vi "Laser Fine Cutting.vi"(0 "configuration file path":path=path "C:/Users/admin/OneDrive/文档/Inlafa.CCV254.MES/System/All Config.ini" caption="配置文件的路径", 1 "fine cutting msic":T1) -> ()   [LabVIEW 2014]
uses:
  Ctl.xio/fine cutting msic ctl.ctl
  SubVIS.xio/DataSocket/DataSocket_Tags.ctl
  Ctl.xio/part type.ctl
  SubVIS.xio/Creat Write List VI's/DefCtrl/Station.ctl
  SubVIS.xio/DataSocket/Write PLC Vars/Write String Var in.vi
  <vilib>/Utility/file.llb/Read From Spreadsheet File (string).vi
  SubVIS.xio/DataSocket/Write PLC Vars/Write Bool Var in.vi
  SubVIS.xio/DataSocket/Read PLC Vars/Read String Var.vi
  SubVIS.xio/DataSocket/Write PLC Vars/Write Dbl Var in.vi
  SubVIS.xio/DataSocket/Read PLC Vars/Read Bool Var.vi
  SubVIS.xio/DataSocket/Read PLC Vars/Read U32 Var.vi
panel:
  in  "SQL information":string
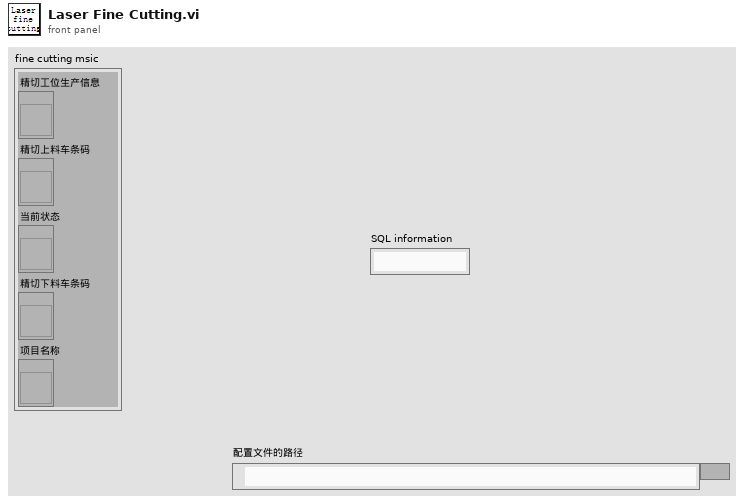
[diagram p1: front panel]
types:
  T1 = cluster{"精切工位生产信息":refnum<vi>, "精切上料车条码":refnum<vi>, "当前状态":refnum<vi>, "精切下料车条码":refnum<vi>, "项目名称":refnum<vi>}
  T2 = typedef "Station.ctl" = enum16{"粗切工位", "热处理工位", "精切工位", "PDF焊接工位", "打凹点预载力工位", "收卷工位", "EOL工位"}
  T3 = typedef "fine cutting msic ctl.ctl" = cluster{"configuration file path":path, "DsOut":T4[], "Hopper in car information":cluster{"Hopper car code":string, "Hopper car No":string, "plate No":string}, "pallet.produced number":i32, "SQL information":string, "Database":string[], "Serial number":i32, "database path":path, "fine cutting msic":cluster{"精切工位生产信息":refnum<vi>, "精切上料车条码":refnum<vi>, "当前状态":refnum<vi>, "精切下料车条码":refnum<vi>, "项目名称":refnum<vi>}, "part type":T5, "scanner1 coms or ip":string, "scanner2 coms or ip":string, "scanner1 resource name out":refnum<visa-resource-name>, "scanner2 resource name out":refnum<visa-resource-name>, "BarCode1":string, "BarCode2":string, "Hopper out information":cluster{"Hopper car code":string, "Hopper car No":string, "plate No":string}, "scanner1 ip ID":refnum<k5>, "scanner2 ip ID":refnum<k5>, "Number of scans":i32}
  T4 = typedef "DataSocket_Tags.ctl" = cluster{"Ds ID":refnum<k13>, "Tag":string}
  T5 = typedef "part type.ctl" = cluster{"项目号":string, "物料代码":string, "零件号":string, "供应商编码":string, "产线编码":string, "客户代码":string, "颜色代码":string, "托盘上限":i32, "加热温度":string, "加热时长":string, "EOL Stations":string}
  T6 = cluster{"Hopper car code":string, "Hopper car No":string, "plate No":string}
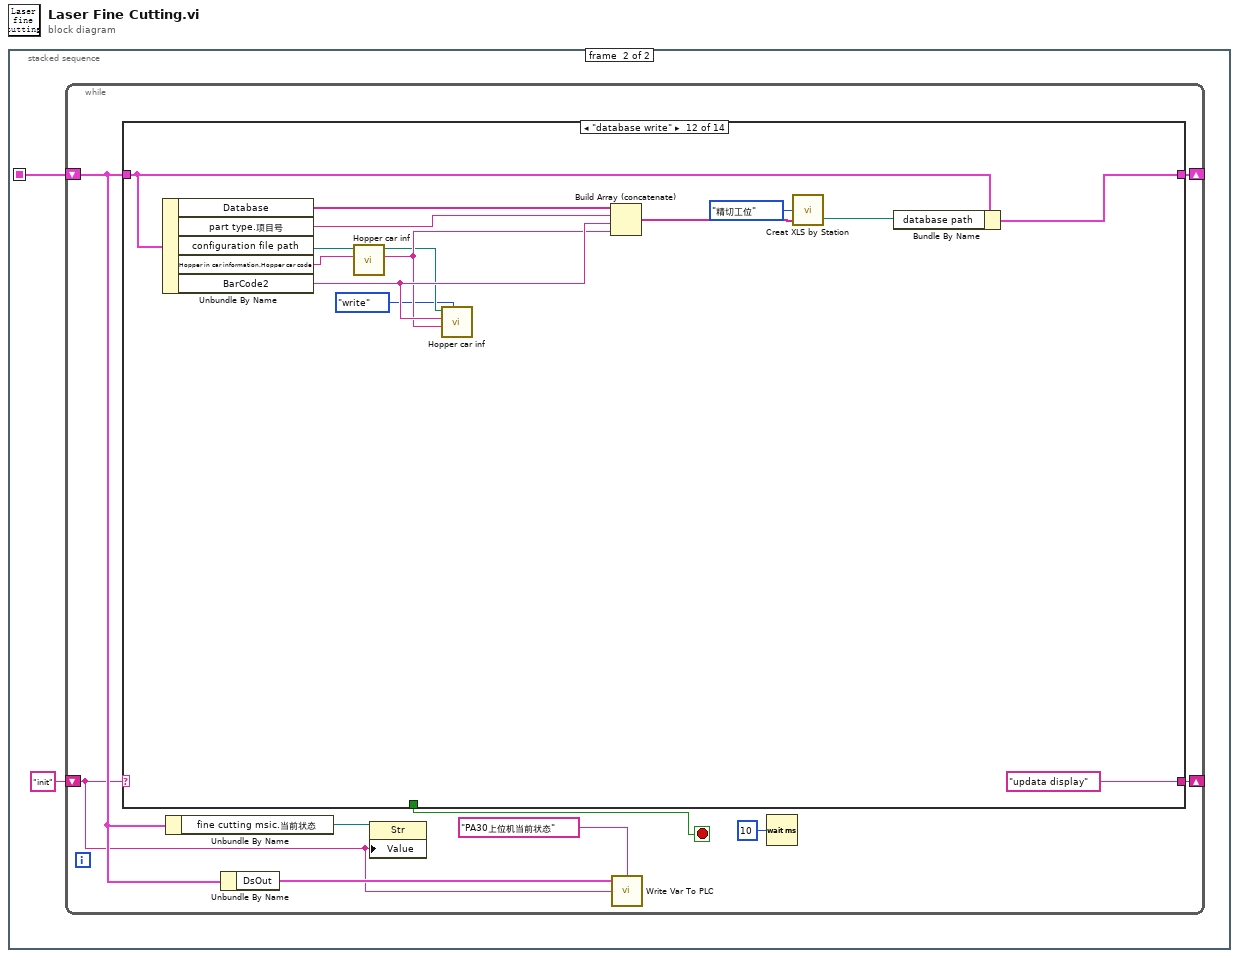
[diagram p0: block diagram]
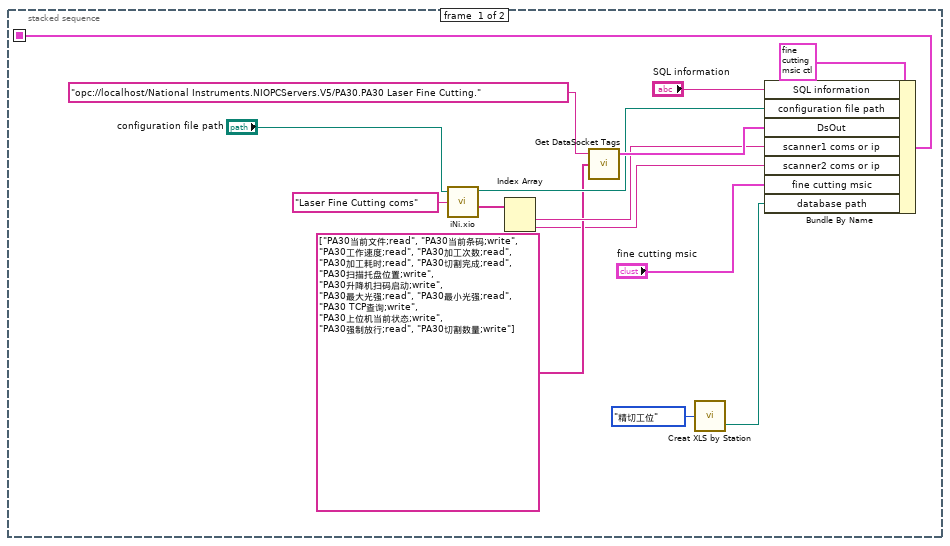
[diagram p2: hidden frame]
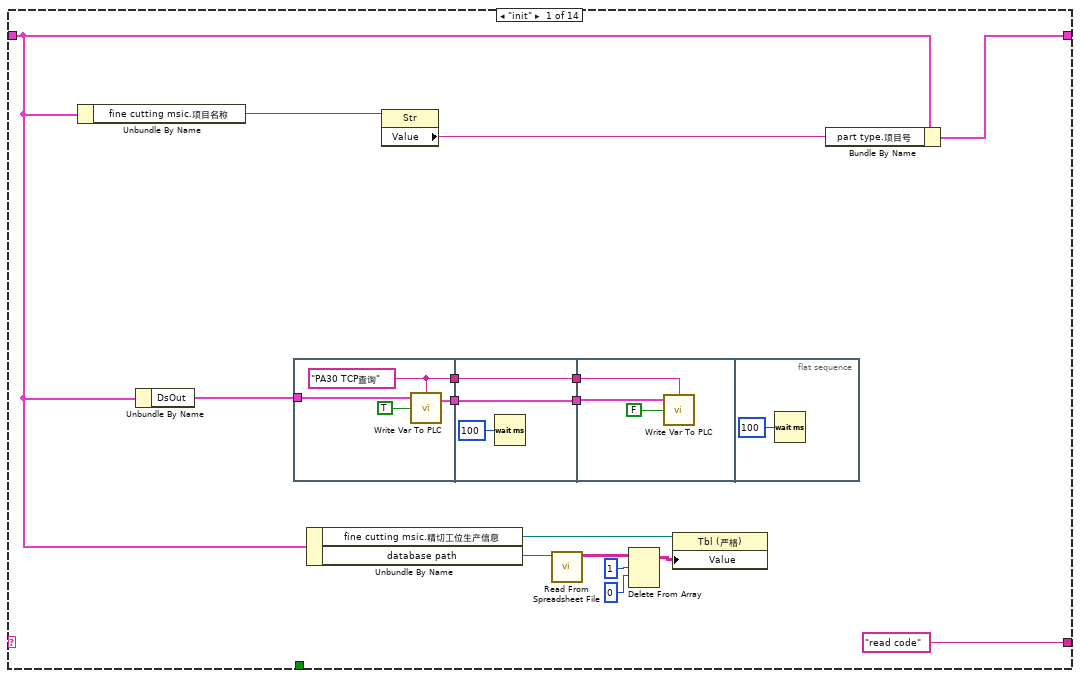
[diagram p3: hidden frame]
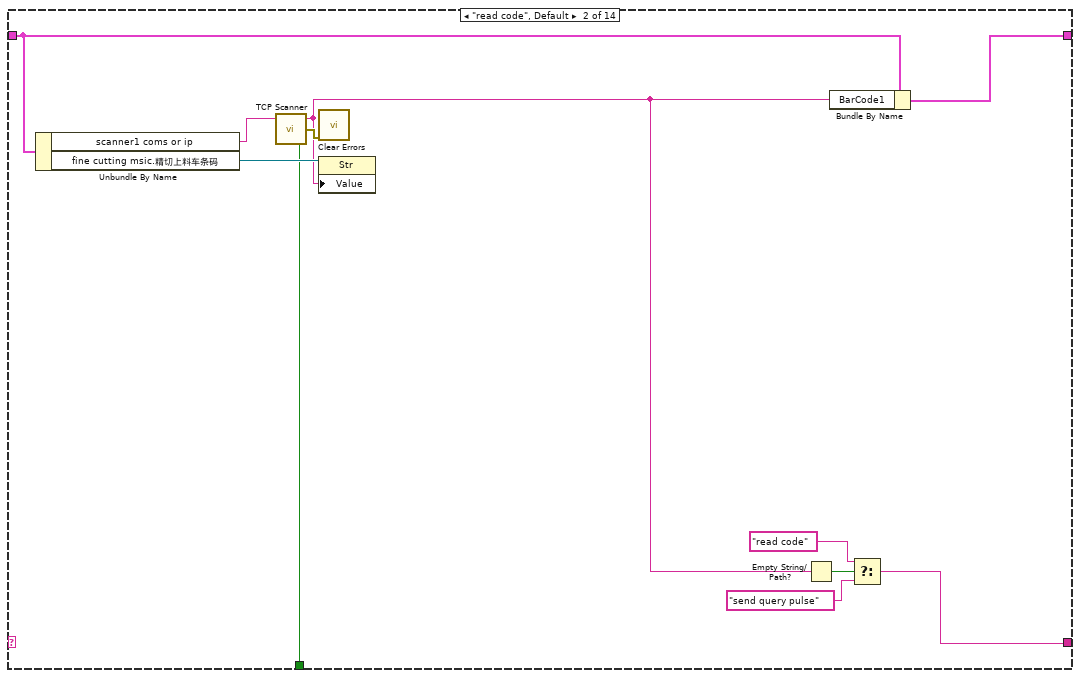
[diagram p4: hidden frame]
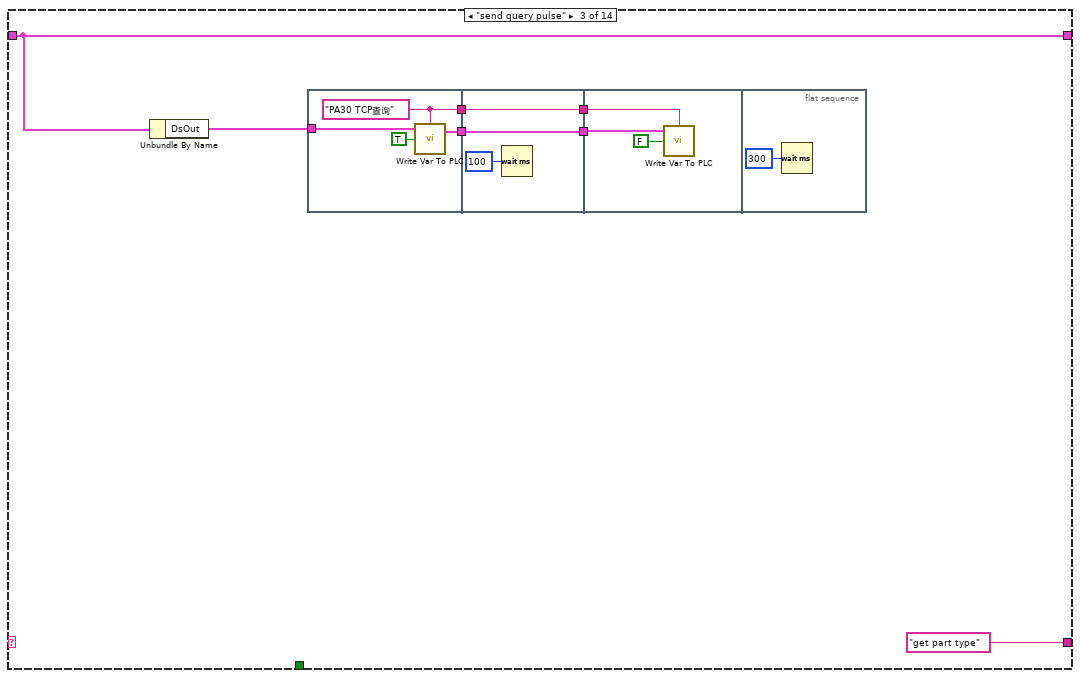
[diagram p5: hidden frame]
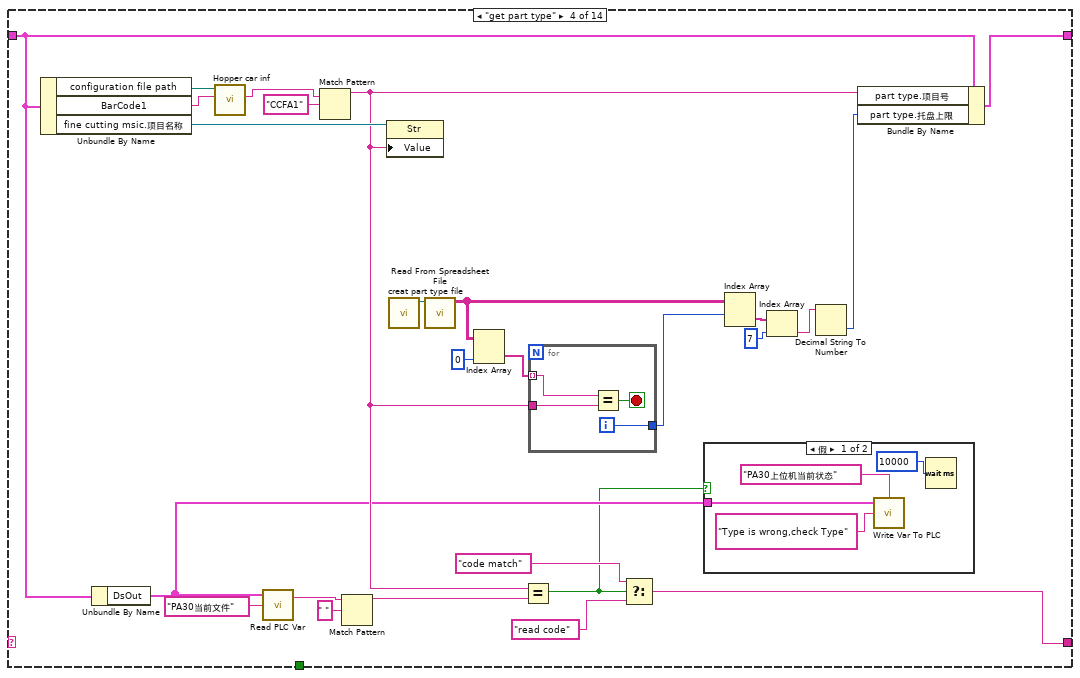
[diagram p6: hidden frame]
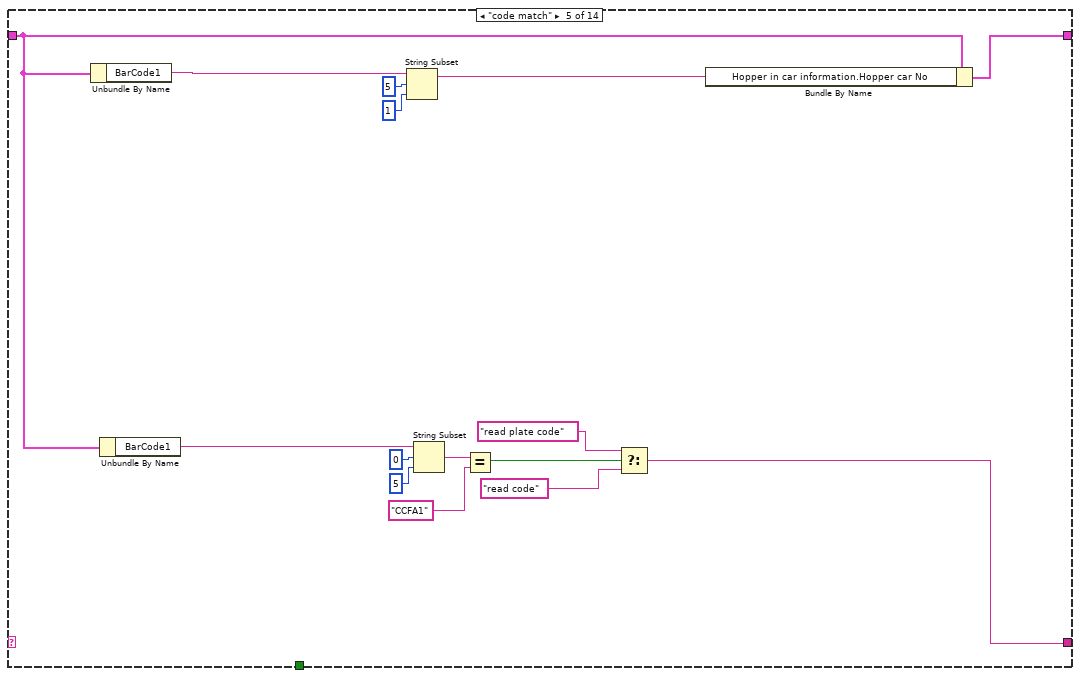
[diagram p8: hidden frame]
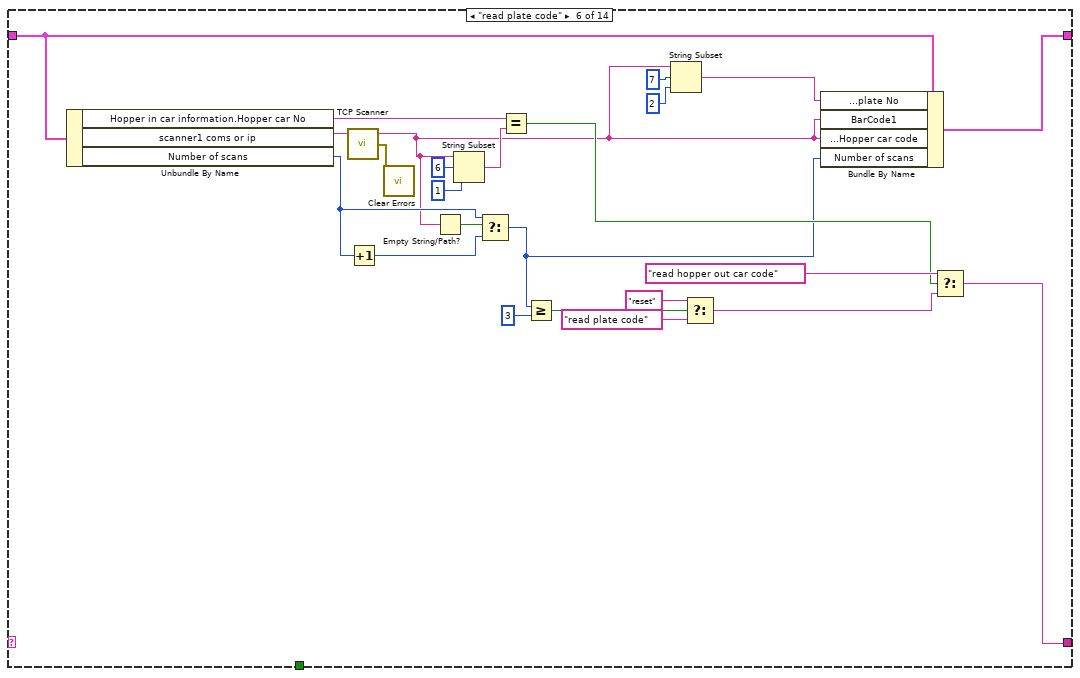
[diagram p9: hidden frame]
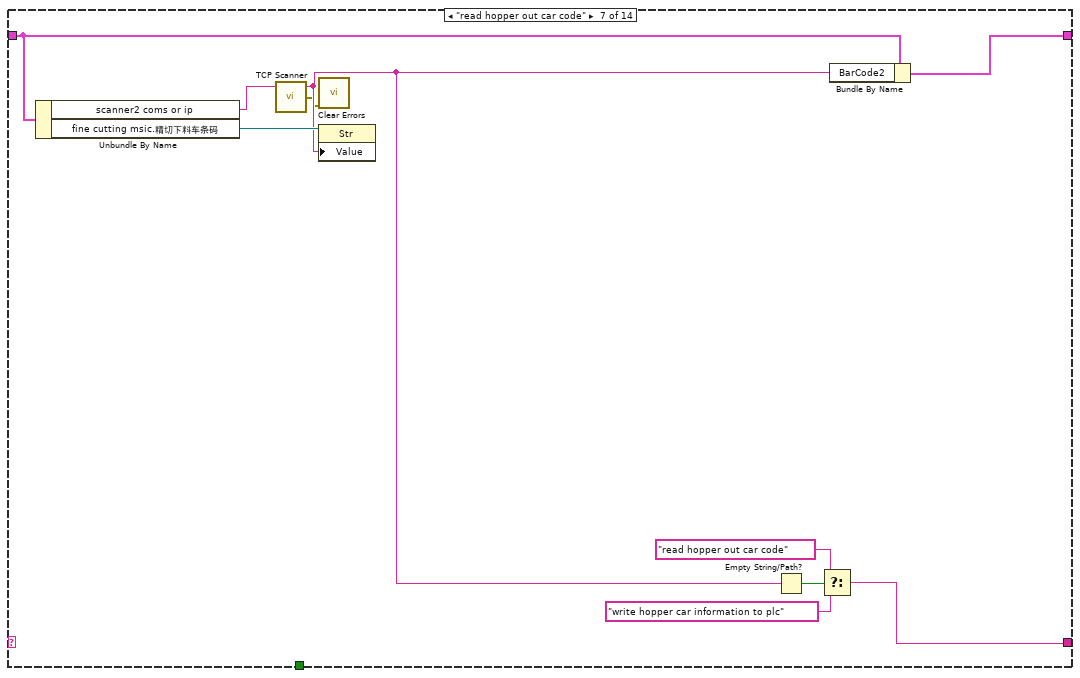
[diagram p10: hidden frame]
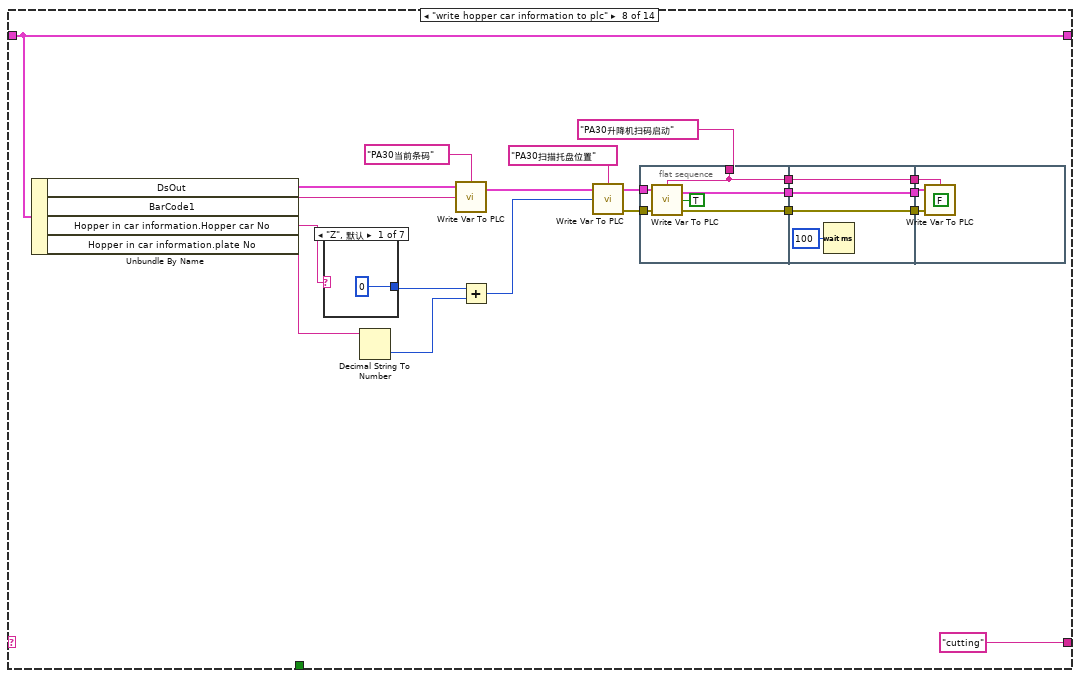
[diagram p11: hidden frame]
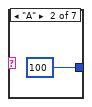
[diagram p12: hidden frame]
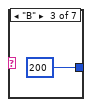
[diagram p13: hidden frame]
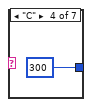
[diagram p14: hidden frame]
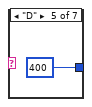
[diagram p15: hidden frame]
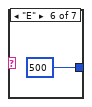
[diagram p16: hidden frame]
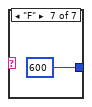
[diagram p17: hidden frame]
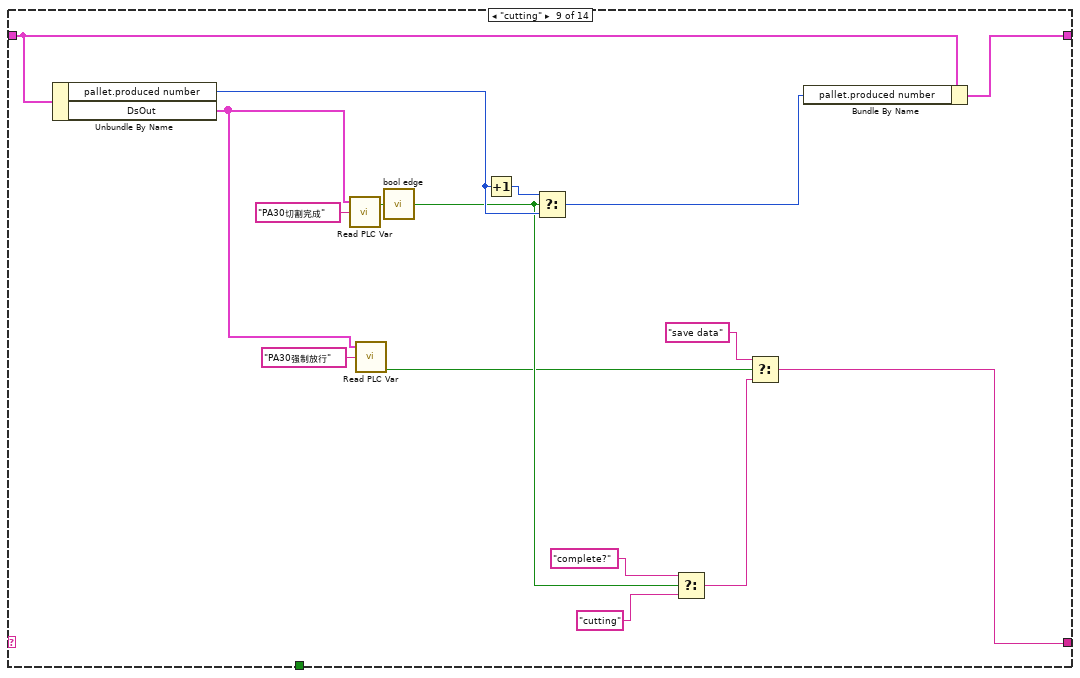
[diagram p18: hidden frame]
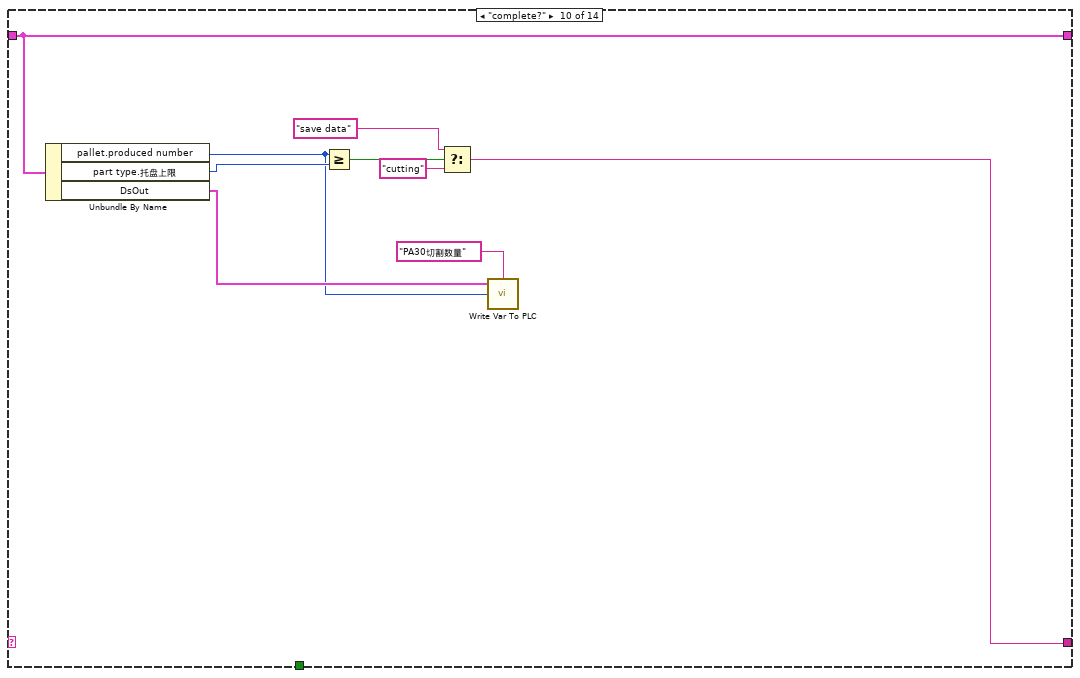
[diagram p19: hidden frame]
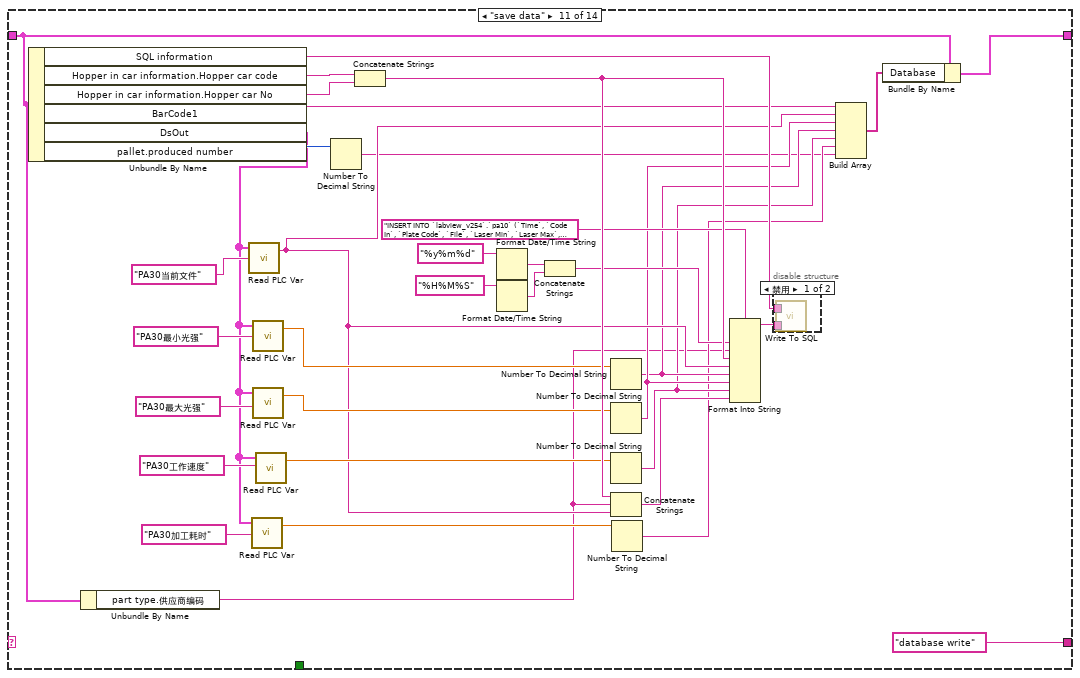
[diagram p20: hidden frame]
diagram:
  n1 = stacked-sequence {
    seq-local: [w3 _] -> [_ w16]
    frame #0 {
      n2 = call "iNi.xio.vi"("configuration file path"="configuration file path", "Sections"="Laser Fine Cutting coms") -> ("configuration file path"=w14:path, "Values"=w12:string[])  [unwired: 1 in, 3 out]
      n3 = Index Array(array=w12) -> (element #1=w11:string, element #2=w5:string)  [unwired: 2 in]
      n4 = call "Get DataSocket Tags.vi"("All Tags"=string[] ["PA30当前文件;read", "PA30当前条码;write", "PA30工作速度;read", "PA30加工次数;read", "PA30加工耗时;read", "PA30切割完成;read", "PA30扫描托盘位置;write", "PA30升降机扫码启动;write", "PA30最大光强;read", "PA30最小光强;read", "PA30 TCP查询;write", "PA30上位机当前状态;write", "PA30强制放行;read", "PA30切割数量;write"], "URL"="opc://localhost/National Instruments.NIOPCServers.V5/PA30.PA30 Laser Fine Cutting.") -> ("DsOut"=w15:T4[])  [unwired: 3 in]
      n5 = call "Creat XLS by Station.vi"("staiton"=Station."精切工位") -> ("new file path (Not A Path if cancelled)"=w2:path)  [unwired: 5 in]
      n6 = Bundle By Name(cluster=T3 {"configuration file path"=path "", "DsOut"=[], "Hopper in car information"={"Hopper car code"="", "Hopper car No"="", "plate No"=""}, "pallet.produced number"=0, "SQL information"="", "Database"=[], "Serial number"=0, "database path"=path "", "fine cutting msic"={"精切工位生产信息"=refnum, "精切上料车条码"=refnum, "当前状态"=refnum, "精切下料车条码"=refnum, "项目名称"=refnum}, "part type"={"项目号"="", "物料代码"="", "零件号"="", "供应商编码"="", "产线编码"="", "客户代码"="", "颜色代码"="", "托盘上限"=0, "加热温度"="", "加热时长"="", "EOL Stations"=""}, "scanner1 coms or ip"="", "scanner2 coms or ip"="", "scanner1 resource name out"="", "scanner2 resource name out"="", "BarCode1"="", "BarCode2"="", "Hopper out information"={"Hopper car code"="", "Hopper car No"="", "plate No"=""}, "scanner1 ip ID"=refnum, "scanner2 ip ID"=refnum, "Number of scans"=0} ("rough cutting msic"), "SQL information"="SQL information", "configuration file path"=w14, "DsOut"=w15, "scanner1 coms or ip"=w11, "scanner2 coms or ip"=w5, "fine cutting msic"="fine cutting msic", "database path"=w2) -> (w3:T3)
    }
    frame #1 {
      n7 = while {
        shift-right: [w26] -> _
        shift-left: w16 -> [w21]
        shift-right: [w25] -> _
        shift-left: "init" ("event") -> [w19]
        stop <- w18 stop-if-true
        n8 = case shown="\"database write\"" w19 {
          tunnel: w21 -> [w27 w62 w66 w90 w119 w144 w163 w166 w219 w227 w234 w281 w288 w296]
          tunnel: [w42 w64 w66 w108 w127 w141 w165 w166 w221 w227 w239 w282 w288 w301] -> w26
          tunnel: ["read code" w56 "get part type" ("f") w89 w125 w142 w158 "cutting" ("event") w208 w230 "database write" ("f") "updata display" ("f") "reset" ("f") "read code" ("f")] -> w25
          tunnel: [_ w54 _ _ _ _ _ _ _ _ _ _ _ _] -> w18
          frame "init" {
            n9 = Unbundle By Name(w27) -> ("fine cutting msic.项目名称"=w40:refnum<vi>)
            n10 = Unbundle By Name(w27) -> ("DsOut"=w34:T4[])
            n11 = flat-sequence {
              tunnel: w34 -> [w46]
              tunnel: [w44] -> w38
              tunnel: [w43] -> w37
              tunnel: w38 -> [w48]
              tunnel: [w48] -> w36
              tunnel: w37 -> [w47]
              tunnel: [w47] -> w35
              tunnel: w36 -> [w52]
              tunnel: w35 -> [w50]
              frame #0 {
                w43 = "PA30 TCP查询" ("Tag IN")
                n12 = call-poly "Write Var To PLC.vi"("Tag IN"=w43, "Bool Var in"=TRUE, "Ds PLCTags IN"=w46) -> ("Ds PLCTags OUT"=w44:T4[])  [unwired: 1 in, 1 out]
              }
              frame #1 {
                n13 = Wait (ms)(milliseconds to wait=u32 100 ("等待时间（毫秒）")) -> ()  [unwired: 1 out]
              }
              frame #2 {
                n14 = call-poly "Write Var To PLC.vi"("Tag IN"=w50, "Bool Var in"=FALSE, "Ds PLCTags IN"=w52) -> ()  [unwired: 1 in, 2 out]
              }
              frame #3 {
                n15 = Wait (ms)(milliseconds to wait=u32 100 ("等待时间（毫秒）")) -> ()  [unwired: 1 out]
              }
            }
            n16 = Unbundle By Name(w27) -> ("fine cutting msic.精切工位生产信息"=w33:refnum<vi>, "database path"=w32:path)
            n17 = property class="Str"(reference=w40) -> ("Value"=w39:string)  [unwired: 1 in, 2 out]
            n18 = call-poly <vilib>:"Read From Spreadsheet File.vi"("file path (dialog if empty)"=w32) -> ("all rows"=w31:string[][])  [unwired: 6 in, 4 out]
            n19 = Delete From Array(array=w31, length=1 ("长度"), index (row)=0 ("索引 (行)")) -> (array with subset deleted=w28:string[][])  [unwired: 1 in, 1 out]
            n20 = property class="Tbl (严格)"(reference=w33, "Value"=w28) -> ()  [unwired: 1 in, 2 out]
            n21 = Bundle By Name(cluster=w27, "part type.项目号"=w39) -> (w42:T3)
          }
          frame "read code", Default {
            n22 = Unbundle By Name(w62) -> ("scanner1 coms or ip"=w61:string, "fine cutting msic.精切上料车条码"=w63:refnum<vi>)
            n23 = call "TCP Scanner.vi"("ip"=w61) -> ("status"=w54:bool, "错误输出"=w60:errorcluster, "Barcode"=w55:string)  [unwired: 2 in]
            n24 = call <vilib>:"Clear Errors.vi"("error in (no error)"=w60) -> ()  [unwired: 5 in, 2 out]
            n25 = property class="Str"(reference=w63, "Value"=w55) -> ()  [unwired: 1 in, 2 out]
            n26 = Empty String/Path?(string/path=w55) -> (empty?=w59:bool)
            n27 = Bundle By Name(cluster=w62, "BarCode1"=w55) -> (w64:T3)
            n28 = Select(t="read code", s=w59, f="send query pulse") -> (s? t:f=w56:string)
          }
          frame "send query pulse" {
            n29 = Unbundle By Name(w66) -> ("DsOut"=w67:T4[])
            n30 = flat-sequence {
              tunnel: w67 -> [w75]
              tunnel: [w73] -> w71
              tunnel: [w72] -> w70
              tunnel: w71 -> [w77]
              tunnel: [w77] -> w69
              tunnel: w70 -> [w76]
              tunnel: [w76] -> w68
              tunnel: w69 -> [w81]
              tunnel: w68 -> [w79]
              frame #0 {
                w72 = "PA30 TCP查询" ("Tag IN")
                n31 = call-poly "Write Var To PLC.vi"("Tag IN"=w72, "Bool Var in"=TRUE, "Ds PLCTags IN"=w75) -> ("Ds PLCTags OUT"=w73:T4[])  [unwired: 1 in, 1 out]
              }
              frame #1 {
                n32 = Wait (ms)(milliseconds to wait=u32 100 ("等待时间（毫秒）")) -> ()  [unwired: 1 out]
              }
              frame #2 {
                n33 = call-poly "Write Var To PLC.vi"("Tag IN"=w79, "Bool Var in"=FALSE, "Ds PLCTags IN"=w81) -> ()  [unwired: 1 in, 2 out]
              }
              frame #3 {
                n34 = Wait (ms)(milliseconds to wait=u32 300 ("等待时间（毫秒）")) -> ()  [unwired: 1 out]
              }
            }
          }
          frame "get part type" {
            n35 = Unbundle By Name(w90) -> ("configuration file path"=w98:path, "BarCode1"=w97:string, "fine cutting msic.项目名称"=w96:refnum<vi>)
            n36 = Unbundle By Name(w90) -> ("DsOut"=w84:T4[])
            n37 = call "Hopper car inf.vi"("key"=w97, "path in"=w98) -> ("value out"=w95:string)  [unwired: 8 in, 1 out]
            n38 = call-poly "Read PLC Var.vi"("Tag IN"="PA30当前文件", "Ds PLCTags IN"=w84) -> ("String Var out"=w87:string)  [unwired: 1 in, 1 out]
            n39 = Match Pattern(string=w95, regular expression="CCFA1" ("正则表达式")) -> (before substring=w88:string)  [unwired: 1 in, 3 out]
            n40 = Match Pattern(string=w87, regular expression=" " ("正则表达式")) -> (before substring=w85:string)  [unwired: 1 in, 3 out]
            n41 = property class="Str"(reference=w96, "Value"=w88) -> ()  [unwired: 1 in, 2 out]
            n42 = call "creat part type file.vi"() -> ("new file path (Not A Path if cancelled)"=w99:path)  [unwired: 11 in]
            n43 = call-poly <vilib>:"Read From Spreadsheet File.vi"("file path (dialog if empty)"=w99) -> ("all rows"=w103:string[][])  [unwired: 6 in, 4 out]
            n44 = Index Array(array=w103, index (col)=0 ("禁用的索引 (列)")) -> (element=w104:string[])  [unwired: 1 in]
            n45 = Equal?(x=w88, y=w85) -> (x = y?=w83:bool)
            n46 = for {
              tunnel: w104 -> [w113] mode=indexing
              tunnel: [w115] -> w102
              tunnel: w88 -> [w114]
              i -> [w115]
              stop <- w116 stop-if-true
              n47 = Equal?(x=w113, y=w114) -> (x = y?=w116:bool)
            }
            n48 = Select(t="code match" ("event"), s=w83, f="read code" ("event")) -> (s? t:f=w89:string)
            n49 = case shown="假" w83 {
              tunnel: w84 -> [w112 _]
              frame False {
                n50 = call-poly "Write Var To PLC.vi"("Tag IN"="PA30上位机当前状态", "String Var in"="Type is wrong,check Type", "Ds PLCTags IN"=w112) -> ()  [unwired: 1 in, 2 out]
                n51 = Wait (ms)(milliseconds to wait=u32 10000 ("等待时间（毫秒）")) -> ()  [unwired: 1 out]
              }
              frame True {
              }
            }
            n52 = Index Array(array=w103, index (row)=w102) -> (element=w101:string[])  [unwired: 1 in]
            n53 = Index Array(array=w101, index=7 ("索引")) -> (element=w106:string)
            n54 = Decimal String To Number(string=w106) -> (number=w100:i32)  [unwired: 2 in, 1 out]
            n55 = Bundle By Name(cluster=w90, "part type.项目号"=w88, "part type.托盘上限"=w100) -> (w108:T3)
          }
          frame "code match" {
            n56 = Unbundle By Name(w119) -> ("BarCode1"=w120:string)
            n57 = Unbundle By Name(w119) -> ("BarCode1"=w118:string)
            n58 = String Subset(string=w120, offset (0)=5 ("偏移量(0)"), length (rest)=1 ("长度（剩余）")) -> (substring=w122:string)
            n59 = String Subset(string=w118, offset (0)=0 ("偏移量(0)"), length (rest)=5 ("长度（剩余）")) -> (substring=w123:string)
            n60 = Equal?(x=w123, y="CCFA1") -> (x = y?=w126:bool)
            n61 = Select(t="read plate code" ("event"), s=w126, f="read code" ("event")) -> (s? t:f=w125:string)
            n62 = Bundle By Name(cluster=w119, "Hopper in car information.Hopper car No"=w122) -> (w127:T3)
          }
          frame "read plate code" {
            n63 = Unbundle By Name(w144) -> ("Hopper in car information.Hopper car No"=w152:string, "scanner1 coms or ip"=w155:string, "Number of scans"=w138:i32)
            n64 = call "TCP Scanner.vi"("ip"=w155) -> ("错误输出"=w140:errorcluster, "Barcode"=w132:string)  [unwired: 2 in, 1 out]
            n65 = Increment(x=w138) -> (x+1=w137:i32)
            n66 = call <vilib>:"Clear Errors.vi"("error in (no error)"=w140) -> ()  [unwired: 5 in, 2 out]
            n67 = Empty String/Path?(string/path=w132) -> (empty?=w139:bool)
            n68 = String Subset(string=w132, offset (0)=6 ("偏移量(0)"), length (rest)=1 ("长度（剩余）")) -> (substring=w149:string)
            n69 = Select(t=w138, s=w139, f=w137) -> (s? t:f=w136:i32)
            n70 = Equal?(x=w152, y=w149) -> (x = y?=w150:bool)
            n71 = Greater Or Equal?(x=w136, y=3) -> (x >= y?=w148:bool)
            n72 = String Subset(string=w132, offset (0)=7 ("偏移量(0)"), length (rest)=2 ("长度（剩余）")) -> (substring=w133:string)
            n73 = Select(t="reset" ("event"), s=w148, f="read plate code" ("event")) -> (s? t:f=w145:string)
            n74 = Bundle By Name(cluster=w144, "Hopper in car information.plate No"=w133, "BarCode1"=w132, "Hopper in car information.Hopper car code"=w132, "Number of scans"=w136) -> (w141:T3)
            n75 = Select(t="read hopper out car code" ("event"), s=w150, f=w145) -> (s? t:f=w142:string)
          }
          frame "read hopper out car code" {
            n76 = Unbundle By Name(w163) -> ("scanner2 coms or ip"=w157:string, "fine cutting msic.精切下料车条码"=w164:refnum<vi>)
            n77 = call "TCP Scanner.vi"("ip"=w157) -> ("错误输出"=w156:errorcluster, "Barcode"=w162:string)  [unwired: 2 in, 1 out]
            n78 = call <vilib>:"Clear Errors.vi"("error in (no error)"=w156) -> ()  [unwired: 5 in, 2 out]
            n79 = property class="Str"(reference=w164, "Value"=w162) -> ()  [unwired: 1 in, 2 out]
            n80 = Empty String/Path?(string/path=w162) -> (empty?=w161:bool)
            n81 = Select(t="read hopper out car code" ("f"), s=w161, f="write hopper car information to plc") -> (s? t:f=w158:string)
            n82 = Bundle By Name(cluster=w163, "BarCode2"=w162) -> (w165:T3)
          }
          frame "write hopper car information to plc" {
            n83 = Unbundle By Name(w166) -> ("DsOut"=w169:T4[], "BarCode1"=w168:string, "Hopper in car information.Hopper car No"=w186:string, "Hopper in car information.plate No"=w185:string)
            n84 = case shown="\"Z\", 默认" w186 {
              tunnel: [0 100 200 300 400 500 600] -> w184
              frame "Z", Default {
              }
              frame "A" {
              }
              frame "B" {
              }
              frame "C" {
              }
              frame "D" {
              }
              frame "E" {
              }
              frame "F" {
              }
            }
            n85 = Decimal String To Number(string=w185) -> (number=w183:i32)  [unwired: 2 in, 1 out]
            n86 = call-poly "Write Var To PLC.vi"("Tag IN"="PA30当前条码", "String Var in"=w168, "Ds PLCTags IN"=w169) -> ("Ds PLCTags OUT"=w170:T4[])  [unwired: 1 in, 1 out]
            n87 = Add(x=w184, y=w183) -> (x+y=w181:i32)
            n88 = call-poly "Write Var To PLC.vi"("Tag IN"="PA30扫描托盘位置", "Dbl Var in"=w181, "Ds PLCTags IN"=w170) -> ("error out"=w180:errorcluster, "Ds PLCTags OUT"=w179:T4[])  [unwired: 1 in]
            n89 = flat-sequence {
              tunnel: w180 -> [w192]
              tunnel: w179 -> [w191]
              tunnel: "PA30升降机扫码启动" ("Tag IN") -> [w188]
              tunnel: [w189] -> w175
              tunnel: [w188] -> w174
              tunnel: [w187] -> w172
              tunnel: [w195] -> w176
              tunnel: w175 -> [w195]
              tunnel: w174 -> [w194]
              tunnel: [w194] -> w173
              tunnel: w172 -> [w193]
              tunnel: [w193] -> w171
              tunnel: w176 -> [w200]
              tunnel: w173 -> [w199]
              tunnel: w171 -> [w198]
              frame #0 {
                n90 = call-poly "Write Var To PLC.vi"("Tag IN"=w188, "错误输入（无错误）"=w192, "Bool Var in"=TRUE, "Ds PLCTags IN"=w191) -> ("error out"=w187:errorcluster, "Ds PLCTags OUT"=w189:T4[])
              }
              frame #1 {
                n91 = Wait (ms)(milliseconds to wait=u32 100 ("等待时间（毫秒）")) -> ()  [unwired: 1 out]
              }
              frame #2 {
                n92 = call-poly "Write Var To PLC.vi"("Tag IN"=w199, "错误输入（无错误）"=w198, "Bool Var in"=FALSE, "Ds PLCTags IN"=w200) -> ()  [unwired: 2 out]
              }
            }
          }
          frame "cutting" {
            n93 = Unbundle By Name(w219) -> ("pallet.produced number"=w222:i32, "DsOut"=w212:T4[])
            n94 = call-poly "Read PLC Var.vi"("Tag IN"="PA30切割完成", "Ds PLCTags IN"=w212) -> ("Bool Var out"=w214:bool)  [unwired: 1 in, 1 out]
            n95 = call-poly "Read PLC Var.vi"("Tag IN"="PA30强制放行", "Ds PLCTags IN"=w212) -> ("Bool Var out"=w211:bool)  [unwired: 1 in, 1 out]
            n96 = call "bool edge.vi"("bool in"=w214) -> ("true-false"=w218:bool)  [unwired: 6 in, 1 out]
            n97 = Increment(x=w222) -> (x+1=w223:i32)
            n98 = Select(t=w223, s=w218, f=w222) -> (s? t:f=w220:i32)
            n99 = Select(t="complete?" ("event"), s=w218, f="cutting" ("event")) -> (s? t:f=w209:string)
            n100 = Select(t="save data" ("event"), s=w211, f=w209) -> (s? t:f=w208:string)
            n101 = Bundle By Name(cluster=w219, "pallet.produced number"=w220) -> (w221:T3)
          }
          frame "complete?" {
            n102 = Unbundle By Name(w227) -> ("pallet.produced number"=w224:i32, "part type.托盘上限"=w232:i32, "DsOut"=w225:T4[])
            n103 = Greater Or Equal?(x=w224, y=w232) -> (x >= y?=w231:bool)
            n104 = Select(t="save data" ("event"), s=w231, f="cutting") -> (s? t:f=w230:string)
            n105 = call-poly "Write Var To PLC.vi"("Tag IN"="PA30切割数量", "Dbl Var in"=w224, "Ds PLCTags IN"=w225) -> ()  [unwired: 1 in, 2 out]
          }
          frame "save data" {
            n106 = Unbundle By Name(w234) -> ("SQL information"=w249:string, "Hopper in car information.Hopper car code"=w251:string, "Hopper in car information.Hopper car No"=w250:string, "BarCode1"=w236:string, "DsOut"=w235:T4[], "pallet.produced number"=w238:i32)
            n107 = Unbundle By Name(w234) -> ("part type.供应商编码"=w233:string)
            n108 = call-poly "Read PLC Var.vi"("Tag IN"="PA30当前文件", "Ds PLCTags IN"=w235) -> ("String Var out"=w247:string)  [unwired: 1 in, 1 out]
            n109 = call-poly "Read PLC Var.vi"("Tag IN"="PA30加工耗时", "Ds PLCTags IN"=w235) -> ("U32 Var out"=w242:dbl)  [unwired: 1 in, 1 out]
            n110 = call-poly "Read PLC Var.vi"("Tag IN"="PA30最小光强", "Ds PLCTags IN"=w235) -> ("U32 Var out"=w256:dbl)  [unwired: 1 in, 1 out]
            n111 = call-poly "Read PLC Var.vi"("Tag IN"="PA30最大光强", "Ds PLCTags IN"=w235) -> ("U32 Var out"=w254:dbl)  [unwired: 1 in, 1 out]
            n112 = call-poly "Read PLC Var.vi"("Tag IN"="PA30工作速度", "Ds PLCTags IN"=w235) -> ("U32 Var out"=w252:dbl)  [unwired: 1 in, 1 out]
            n113 = Number To Decimal String(number=w238) -> (decimal integer string=w237:string)  [unwired: 1 in]
            n114 = Concatenate Strings(w251, w250) -> (w267:string)
            n115 = Format Date/Time String(time format string (%c)="%y%m%d" ("时间格式字符串(%c)")) -> (date/time string=w262:string)  [unwired: 2 in]
            n116 = Format Date/Time String(time format string (%c)="%H%M%S" ("时间格式字符串(%c)")) -> (date/time string=w261:string)  [unwired: 2 in]
            n117 = Concatenate Strings(w262, w261) -> (w259:string)
            n118 = Number To Decimal String(number=w256) -> (decimal integer string=w245:string)  [unwired: 1 in]
            n119 = Number To Decimal String(number=w254) -> (decimal integer string=w246:string)  [unwired: 1 in]
            n120 = Number To Decimal String(number=w252) -> (decimal integer string=w244:string)  [unwired: 1 in]
            n121 = Concatenate Strings(w267, w233, w247) -> (w264:string)
            n122 = Number To Decimal String(number=w242) -> (decimal integer string=w241:string)  [unwired: 1 in]
            n123 = Format Into String(format string="INSERT INTO `labview_v254`.`pa10` (`Time`, `Code In`, `Plate Code`, `File`, `Laser Min`, `Laser Max`, `Vel`, `Code Out`) VALUES ('%s', '%s', '%s', '%s', '%s', '%s', '%s', '%s');", w259, w233, w267, w247, w245, w246, w244, w264) -> (resulting string=w265:string)  [unwired: 2 in, 1 out]
            n124 = disable-structure shown="禁用" {
              disable-tunnel: w265 -> [w269 _]
              disable-tunnel: w249 -> [w268 _]
              frame Disabled {
                n125 = call "Write To SQL.vi"("SQL query"=w269, "connection information"=w268) -> ()  [unwired: 1 out]
              }
              frame Enabled {
              }
            }
            n126 = Build Array(w236, w247, w246, w245, w244, w241, w237) -> (w240:string[])
            n127 = Bundle By Name(cluster=w234, "Database"=w240) -> (w239:T3)
          }
          frame "database write" {
            n128 = Unbundle By Name(w281) -> ("Database"=w280:string[], "part type.项目号"=w279:string, "configuration file path"=w278:path, "Hopper in car information.Hopper car code"=w277:string, "BarCode2"=w276:string)
            n129 = call "Hopper car inf.vi"("key"=w277, "path in"=w278) -> ("value out"=w275:string, "path out"=w274:path)  [unwired: 8 in]
            n130 = call "Hopper car inf.vi"("write\\read（read)"=enum16{"read", "write"}."write" ("write\\read（read)"), "value"=w275, "key"=w276, "path in"=w274) -> ()  [unwired: 6 in, 2 out]
            n131 = Build Array (concatenate)(w280, w279, w276, w275) -> (w271:string[])
            n132 = call "Creat XLS by Station.vi"("staiton"=Station."精切工位", "data in"=w271) -> ("new file path (Not A Path if cancelled)"=w272:path)  [unwired: 4 in]
            n133 = Bundle By Name(cluster=w281, "database path"=w272) -> (w282:T3)
          }
          frame "updata display" {
            n134 = Unbundle By Name(w288) -> ("fine cutting msic.精切工位生产信息"=w290:refnum<vi>, "database path"=w289:path)
            n135 = call-poly <vilib>:"Read From Spreadsheet File.vi"("file path (dialog if empty)"=w289) -> ("all rows"=w287:string[][])  [unwired: 6 in, 4 out]
            n136 = Delete From Array(array=w287, length=1 ("长度"), index (row)=0 ("索引 (行)")) -> (array with subset deleted=w284:string[][])  [unwired: 1 in, 1 out]
            n137 = property class="Tbl (严格)"(reference=w290, "Value"=w284) -> ()  [unwired: 1 in, 2 out]
          }
          frame "reset" {
            w293 = ""
            w297 = "" ("BarCode")
            n138 = Unbundle By Name(w296) -> ("fine cutting msic.精切上料车条码"=w295:refnum<vi>, "fine cutting msic.精切下料车条码"=w294:refnum<vi>)
            n139 = property class="Str"(reference=w295, "Value"=w293) -> ()  [unwired: 1 in, 2 out]
            n140 = property class="Str"(reference=w294, "Value"=w293) -> ()  [unwired: 1 in, 2 out]
            n141 = Bundle By Name(cluster=w296, "Number of scans"=0, "pallet.produced number"=0, "BarCode1"=w297, "BarCode2"=w297, "Database"=string[] [], "Hopper in car information"=T6 {"Hopper car code"="", "Hopper car No"="", "plate No"=""} ("Hopper car information")) -> (w301:T3)
          }
        }
        n142 = Unbundle By Name(w21) -> ("fine cutting msic.当前状态"=w23:refnum<vi>)
        n143 = Unbundle By Name(w21) -> ("DsOut"=w20:T4[])
        n144 = property class="Str"(reference=w23, "Value"=w19) -> ()  [unwired: 1 in, 2 out]
        n145 = call-poly "Write Var To PLC.vi"("Tag IN"="PA30上位机当前状态", "String Var in"=w19, "Ds PLCTags IN"=w20) -> ()  [unwired: 1 in, 2 out]
        n146 = Wait (ms)(milliseconds to wait=u32 10 ("等待时间（毫秒）")) -> ()  [unwired: 1 out]
      }
    }
  }
